vi "Fetch Multi Eval Meas Trace SEM RBW Results.vi"(7 "Resolution BW (1000 kHz)":T1=1 items=["120 kHz", "1000 kHz"], 8 "error in (no error)":errorcluster, 9 "Result Type (Current)":i32(ring) items=["Current"=0, "Average"=1, "Maximum"=4], 10 "Instance (1)":T2=1, 11 "VISA resource name":refnum<visa-resource-name>) -> (0 "error out":errorcluster, 1 "Trace SEM RBW Results":dbl[](array[numeric]) format="%^.3e", 2 "Reliability":i32, 3 "VISA resource name out":refnum<visa-resource-name>)   [LabVIEW 2020, in "Rohde&Schwarz CMXP NR FR2 Measurement.lvlib"]
doc: "Returns the values of the spectrum emission traces. Separate traces are available for the individual resolution bandwidths (<kHz>).\n\nAttributes:\nRSCMXPNRFR2M_ATTR_FETCH_MULTI_EVAL_MEASUREMENT_SEM_TRACE_RBW_AVERAGE_RESULTS\nRSCMXPNRFR2M_ATTR_FETCH_MULTI_EVAL_MEASUREMENT_SEM_TRACE_RBW_CURRENT_RESULTS\nRSCMXPNRFR2M_ATTR_FETCH_MULTI_EVAL_MEASUREMENT_SEM_TRACE_RBW_MAXIMUM_RESULTS\n\nRemote-control commands:\nFETCh:NRMMw:MEAS<i>:MEValuation:TRACe:SEMask:RBW<kHz>:AVERage?\nFETCh:NRMMw:MEAS<i>:MEValuation:TRACe:SEMask:RBW<kHz>:CURRent?\nFETCh:NRMMw:MEAS<i>:MEValuation:TRACe:SEMask:RBW<kHz>:MAXimum?"
uses:
  <instrlib>/Rohde&Schwarz CMXP NR FR2 Measurement/Rohde&Schwarz CMXP NR FR2 Measurement.lvlib
  <instrlib>/Rohde&Schwarz CMXP NR FR2 Measurement/Private/_Instance.ctl
  <instrlib>/Rohde&Schwarz CMXP NR FR2 Measurement/Private/_Resolution BW.ctl
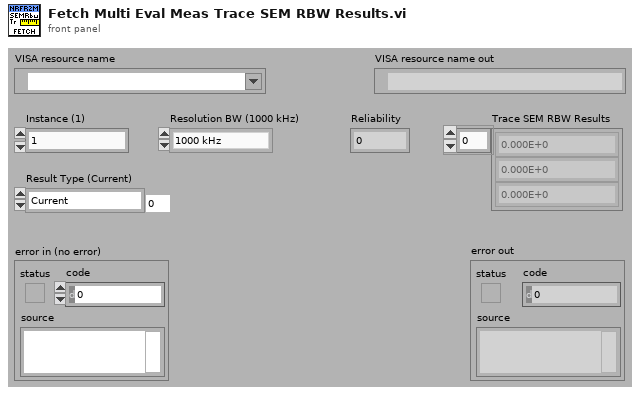
[diagram p1: front panel]
types:
  T1 = typedef "Rohde&Schwarz CMXP NR FR2 Measurement.lvlib/_Resolution BW.ctl" = i32
  T2 = typedef "Rohde&Schwarz CMXP NR FR2 Measurement.lvlib/_Instance.ctl" = i32
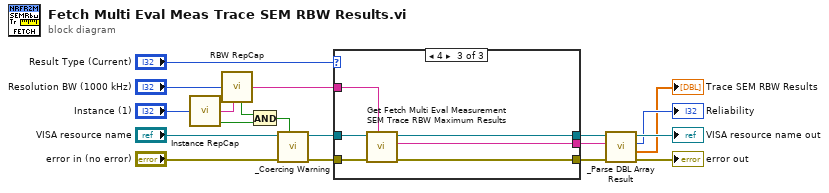
[diagram p0: block diagram]
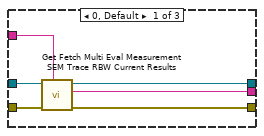
[diagram p2: hidden frame]
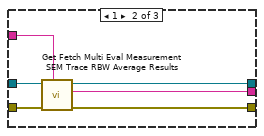
[diagram p3: hidden frame]
diagram:
  n1 = call <instrlib>:"Instance RepCap.vi"("Instance In"="Instance (1)") -> ("In Range?"=w18:bool, "RepCap Identifier Out"=w1:string)  [unwired: 1 in]
  n2 = call <instrlib>:"RBW RepCap.vi"("RBW In"="Resolution BW (1000 kHz)", "RepCap String In (\"\")"=w1) -> ("In Range?"=w17:bool, "RepCap Identifier Out"=w11:string)
  n3 = And(x=w17, y=w18) -> (x .and. y?=w19:bool)
  n4 = call <instrlib>:"_Coercing Warning.vi"("In Range?"=w19, "error in (no error)"="error in (no error)", "VISA resource name"="VISA resource name") -> ("error out"=w16:errorcluster, "VISA resource name out"=w15:refnum<visa-resource-name>)  [unwired: 7 in]
  n5 = case shown="4" "Result Type (Current)" {
    tunnel: w16 -> [w25 w31 w37]
    tunnel: w15 -> [w24 w30 w36]
    tunnel: [w23 w29 w35] -> w12
    tunnel: [w22 w28 w34] -> w14
    tunnel: [w21 w27 w33] -> w13
    tunnel: w11 -> [w20 w26 w32]
    frame 0, Default {
      n6 = call "Get Fetch Multi Eval Measurement SEM Trace RBW Current Results"("Repeated Capabilities"=w20, "error in (no error)"=w25, "instrument handle"=w24) -> ("error out"=w23:errorcluster, "Fetch Multi Eval Measurement SEM Trace RBW Current Results"=w21:string, "instrument handle out"=w22:refnum<visa-resource-name>)  [unwired: 6 in]
    }
    frame 1 {
      n7 = call "Get Fetch Multi Eval Measurement SEM Trace RBW Average Results"("Repeated Capabilities"=w26, "error in (no error)"=w31, "instrument handle"=w30) -> ("error out"=w29:errorcluster, "Fetch Multi Eval Measurement SEM Trace RBW Average Results"=w27:string, "instrument handle out"=w28:refnum<visa-resource-name>)  [unwired: 6 in]
    }
    frame 4 {
      n8 = call "Get Fetch Multi Eval Measurement SEM Trace RBW Maximum Results"("Repeated Capabilities"=w32, "error in (no error)"=w37, "instrument handle"=w36) -> ("error out"=w35:errorcluster, "Fetch Multi Eval Measurement SEM Trace RBW Maximum Results"=w33:string, "instrument handle out"=w34:refnum<visa-resource-name>)  [unwired: 6 in]
    }
  }
  n9 = call <instrlib>:"_Parse DBL Array Result.vi"("error in (no error)"=w12, "Input String"=w13, "VISA resource name"=w14) -> ("error out"=→"error out":errorcluster, "Results"=→"Trace SEM RBW Results":dbl[], "Reliability"=→"Reliability":i32, "VISA resource name out"=→"VISA resource name out":refnum<visa-resource-name>)  [unwired: 5 in]
